vi "Get Image Delays.vi"(8 "error in (no error)":errorcluster, 10 "frame":u16, 11 "Header in":refnum<class "Header.lvclass">) -> (0 "error out":errorcluster, 3 "Header out":refnum<class "Header.lvclass">)   [LabVIEW 2018, in "Header.lvclass"]
uses:
  Header.lvclass
  C:/Users/observer/Desktop/SPARC4_ACS/SPARC4_ACS/Simulated_Header/Simulated_Header.lvclass
  Simulated_Header/Simulated_Header.lvclass
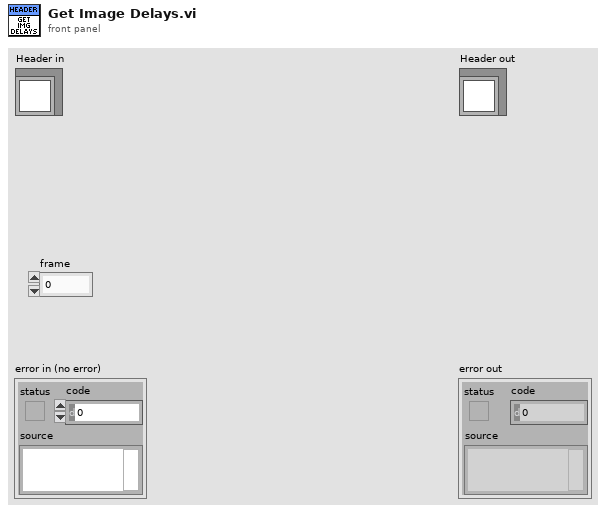
[diagram p1: front panel]
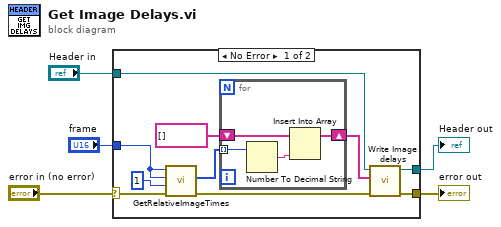
[diagram p0: block diagram]
diagram:
  n1 = case shown="No Error" "error in (no error)" {
    selector: "error in (no error)" -> [w13 w21]
    tunnel: [w8 w21] -> w2
    tunnel: [w10 w20] -> w3
    tunnel: "Header in" -> [w11 w20]
    tunnel: "frame" -> [w6 _]
    frame No Error {
      n2 = call <userlib>:"GetRelativeImageTimes.vi"("error in (no error)"=w13, "size"=u32 1 ("first"), "last"=w6, "first"=w6) -> ("error out"=w9:errorcluster, "arr"=w15:u64[])  [unwired: 5 in, 1 out]
      n3 = for {
        shift-right: [w16] -> w12
        shift-left: string[] [] -> [w17]
        tunnel: w15 -> [w19] mode=indexing
        n4 = Number To Decimal String(number=w19) -> (decimal integer string=w18:string)  [unwired: 1 in]
        n5 = Insert Into Array(array=w17, new element=w18) -> (w16:string[])  [unwired: 1 in]
      }
      n6 = call "Write Image delays.vi"("error in (no error)"=w9, "Image delays"=w12, "Header in"=w11) -> ("error out"=w8:errorcluster, "Header out"=w10:refnum<class "Header.lvclass">)  [unwired: 7 in]
    }
    frame Error {
    }
  }
  "error out" <- w2
  "Header out" <- w3
